vi "PH_Trendviewer_Powermeter.constructor.vi"(0 "name":string, 2 "data in":string, 5 "error in":errorcluster) -> (14 "i ref out":refnum<vi>, 16 "data out":string, 19 "error out":errorcluster)   [LabVIEW 2014, in "PH_Trendviewer_Powermeter.lvlib"]
doc: "author: Stefan Götte, GSI\n\nLicense Agreement for this software:\n\nCopyright (C)\nGesellschaft für Schwerionenforschung, GSI\nPlanckstr. 1\n64291 Darmstadt\nGermany\n\nContact: D.Beck@gsi.de \n\nThis program is free software; you can redistribute it and/or modify it under the terms of the \nGNU General Public License as published by the Free Software Foundation; either version 2 of \nthe license, or (at your option) any later version.\n\nThis program is distributed in the hope that it will be useful, but WITHOUT ANY WARRANTY; \nwithout even the implied warranty of MERCHANTABILITY or FITNESS FOR A PARTICULAR PURPOSE. See the GNU General License for more details (http://www.gnu.org).\n\nGesellschaft für Schwerionenforschung, GSI\nPlanckstr. 1, 64291 Darmstadt, Germany\nFor all questions and ideas contact: M.Richter@gsi.de, H.Brand@gsi.de or D.Beck@gsi.de.\nLast update: 16-JUN-2004"
uses:
  PH_Trendviewer_Powermeter.lvlib
  CSCore/CSObj/CSObj.lvlib
  PH_Class/PH_Class.lvlib
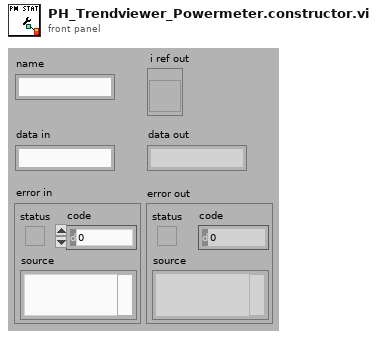
[diagram p1: front panel]
types:
  T1 = enum16{"SetAttribute", "GetAttribute", "CreateAttribute", "DestroyAttribute", "DestroyAllAtributes"}
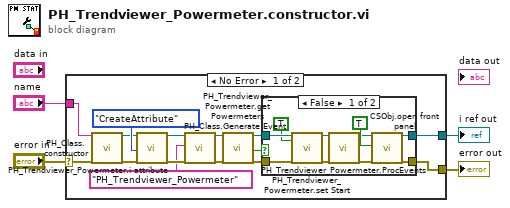
[diagram p0: block diagram]
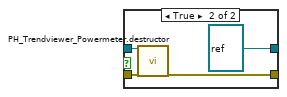
[diagram p2: hidden frame]
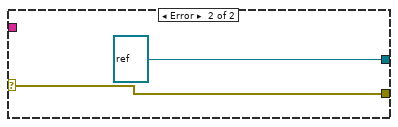
[diagram p3: hidden frame]
diagram:
  n1 = case shown="No Error" "error in" {
    selector: "error in" -> [w12 w35]
    tunnel: "name" -> [w16 _]
    tunnel: [w10 refnum<vi> refnum ("i ref out")] -> w3
    tunnel: [w11 w35] -> w2
    frame No Error {
      n2 = call "PH_Class.constructor.vi"("name"=w16, "error in"=w12) -> ("i ref out"=w18:refnum<vi>, "error out"=w17:errorcluster)  [unwired: 15 in, 1 out]
      n3 = call "PH_Trendviewer_Powermeter.i attribute.vi"("VI Refnum"=w18, "Action"=T1."CreateAttribute", "error in (no error)"=w17) -> ("VI Refnum out"=w15:refnum<vi>, "error out"=w6:errorcluster)  [unwired: 14 in, 1 out]
      n4 = call "PH_Class.Generate Event.vi"("i ref in"=w15, "Class"="PH_Trendviewer_Powermeter", "error in (no error)"=w6) -> ("i ref out"=w14:refnum<vi>, "error out"=w13:errorcluster)  [unwired: 15 in]
      n5 = call "PH_Trendviewer_Powermeter.get Powermeters.vi"("i ref in"=w14, "error in"=w13) -> ("i ref out"=w8:refnum<vi>, "No Powermeter selected?"=w7:bool, "error out"=w9:errorcluster)  [unwired: 15 in]
      n6 = case shown="False" w7 {
        tunnel: [w29 w31] -> w11
        tunnel: [w28 refnum<vi> refnum ("i ref out")] -> w10
        tunnel: w9 -> [w24 w32]
        tunnel: w8 -> [w22 w33]
        frame False {
          n7 = call "PH_Trendviewer_Powermeter.set Start.vi"("i ref in"=w22, "Start"=TRUE, "error in (no error)"=w24) -> ("i ref out"=w21:refnum<vi>, "error out"=w23:errorcluster)  [unwired: 15 in]
          n8 = call "PH_Trendviewer_Powermeter.ProcEvents.vi"("i ref in"=w21, "error in (no error)"=w23) -> ("i ref out"=w25:refnum<vi>, "error out"=w26:errorcluster)  [unwired: 16 in]
          n9 = call "CSObj.open front panel.vi"("i ref in"=w25, "frontPanelOpen"=TRUE ("front panel open"), "error in (no error)"=w26) -> ("i ref out"=w28:refnum<vi>, "error out"=w29:errorcluster)  [unwired: 15 in]
        }
        frame True {
          n10 = call "PH_Trendviewer_Powermeter.destructor.vi"("i ref in"=w33, "error in(no error)"=w32) -> ("error out"=w31:errorcluster)  [unwired: 17 in]
        }
      }
    }
    frame Error {
    }
  }
  "i ref out" <- w3
  "error out" <- w2
